vi "Hardware Updated Event.vi"() -> (3 "Hardware Update Data":refnum<user-event>)   [LabVIEW 2020]
uses:
  Hardware Update Event Data.ctl
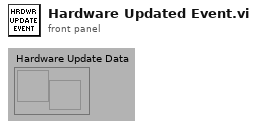
[diagram p1: front panel]
types:
  T1 = typedef "Hardware Update Event Data.ctl" = variant
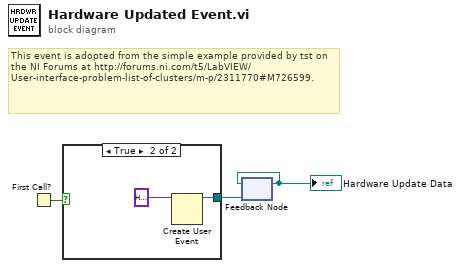
[diagram p0: block diagram]
diagram:
  # "This event is adopted from the simple example provided by tst on the NI Forums at http://forums.ni.com/t5/LabVIEW/User-interface-problem-list-of-clusters/m-p/2311770#M726599."
  n1 = First Call?() -> (First Call?: T/F=w2:bool)
  n2 = case shown="True" w2 {
    tunnel: [_ w5] -> w3
    frame False {
    }
    frame True {
      n3 = Create User Event(user event datatype=T1 variant ("Hardware Update Data")) -> (user event=w5:refnum<user-event>)  [unwired: 1 in, 1 out]
    }
  }
  n4 = feedback #1(w3) -> (w1:refnum<user-event>)
  "Hardware Update Data" <- w1
  n5 = feedback-in #1(w1) -> ()
